vi "From file_test1.vi"() -> (0 "Y subarray":string[](array[string]), 1 "X subarray":string[](array[string]), 2 "Ready?":bool)   [LabVIEW 2021]
uses:
  <vilib>/Utility/file.llb/Read Delimited Spreadsheet (string).vi
panel:
  out "Waveform Graph":dbl[][](graph)
  in  "X data":string(combo)
  out "all rows":string[][](array[string])
  in  "Y data":string(combo)
  in  "Add":bool
  in  "Cancel":bool
  in  "From file (csv)":path caption="file path (dialog if empty)"
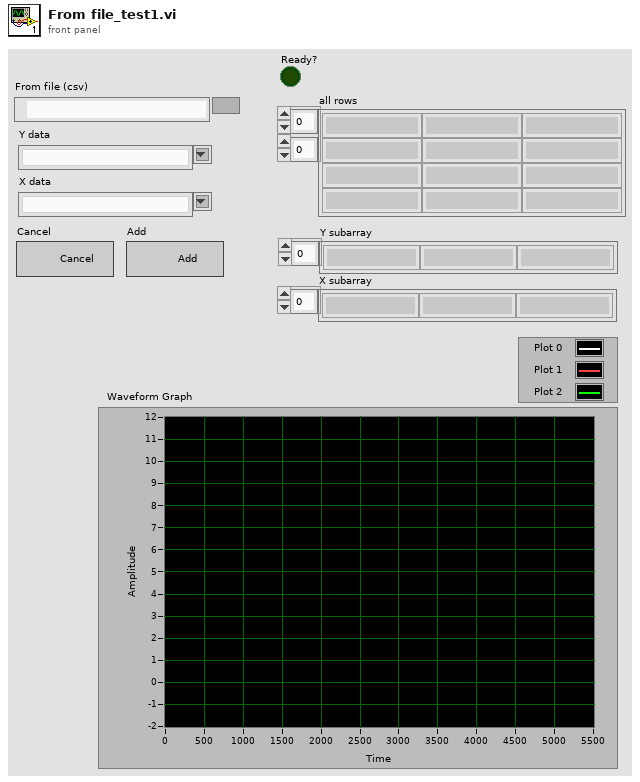
[diagram p1: front panel]
types:
  T1 = enum32{"Invalid", "Standard", "Closed", "Hidden", "Minimized", "Maximized"}
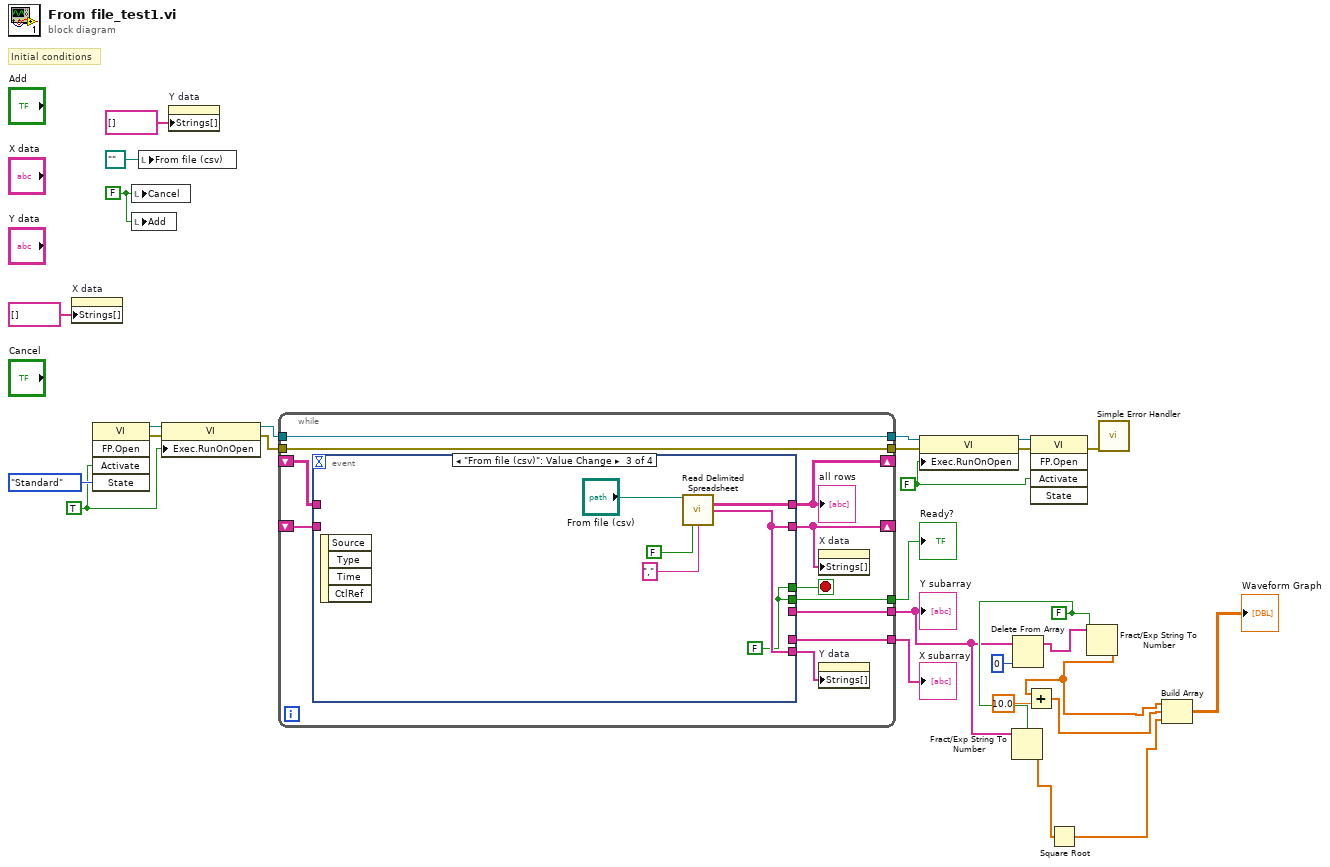
[diagram p0: block diagram]
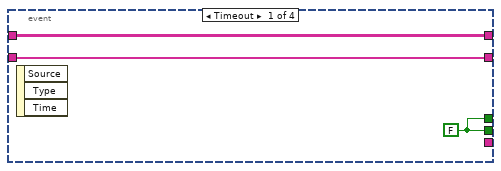
[diagram p2: hidden frame]
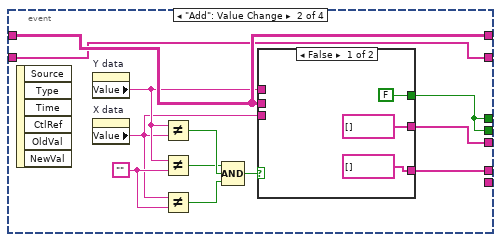
[diagram p3: hidden frame]
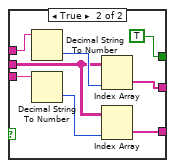
[diagram p4: hidden frame]
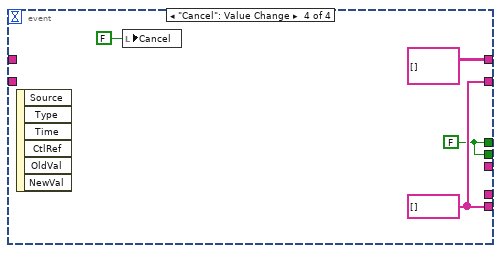
[diagram p5: hidden frame]
diagram:
  w9 = FALSE ("use system decimal point (T)")
  w12 = FALSE ("Activate?")
  w17 = TRUE ("Activate?")
  w27 = FALSE
  # "Initial conditions"
  n1 = property on="X data" class="CmbBox"("Strings[]"=string[] [] ("all rows")) -> ()  [unwired: 2 in, 2 out]
  n2 = invoke class="VI" method="FP.Open"("Activate"=w17, "State"=T1."Standard") -> (reference out=w19:refnum<vi>, error out=w20:errorcluster)  [unwired: 3 in, 3 out]
  n3 = local write "Cancel"(w27) -> ()
  n4 = local write "Add"(w27) -> ()
  n5 = local write "From file (csv)"(path "" ("From file (csv)")) -> ()
  n6 = property class="VI"(reference=w19, error in=w20, "Exec.RunOnOpen"=w17) -> (reference out=w18:refnum<vi>, error out=w21:errorcluster)
  n7 = property on="Y data" class="CmbBox"("Strings[]"=string[] [] ("Strings []")) -> ()  [unwired: 2 in, 2 out]
  n8 = while {
    shift-right: [w36] -> _
    shift-left: _ -> [w38]
    shift-right: [w31] -> _
    shift-left: _ -> [w37]
    tunnel: [w35] -> w1
    tunnel: [w34] -> w5
    tunnel: [w32] -> w26
    tunnel: w21 -> [w29]
    tunnel: w18 -> [w30]
    tunnel: [w30] -> w14
    tunnel: [w29] -> w13
    stop <- w39 stop-if-true
    n9 = event shown="[2] \"From file (csv)\": Value Change" {
      selector: _ -> [_ _ _ _]
      dyn-events: _ -> [_ _ _ _]
      timeout: _ -> [_ _ _ _]
      tunnel: [w42 w49 w68 string[][] [] ("all rows")] -> w36
      tunnel: [w41 w48 w67 w73] -> w31
      tunnel: [w40 w45 w66 w72] -> w39
      tunnel: w38 -> [w42 w49 _ _]
      tunnel: w37 -> [w41 w48 _ _]
      tunnel: [_ w47 _ _] -> w35
      tunnel: [_ w46 _ _] -> w34
      tunnel: [_ _ w67 w73] -> w33
      tunnel: [w40 w45 w66 w72] -> w32
      event Timeout {
        w40 = FALSE
        n10 = event-data() -> ()  [unwired: 1 in, 3 out]
      }
      event "Add": Value Change {
        w51 = ""
        n11 = event-data() -> ()  [unwired: 1 in, 6 out]
        n12 = property on="Y data" class="CmbBox"() -> ("Value"=w44:string)  [unwired: 2 in, 2 out]
        n13 = property on="X data" class="CmbBox"() -> ("Value"=w43:string)  [unwired: 2 in, 2 out]
        n14 = Not Equal?(x=w44, y=w43) -> (x != y?=w53:bool)
        n15 = Not Equal?(x=w44, y=w51) -> (x != y?=w52:bool)
        n16 = Not Equal?(x=w43, y=w51) -> (x != y?=w54:bool)
        n17 = Compound Arithmetic op=AND(w52, w53, w54) -> (w50:bool)
        n18 = case shown="False" w50 {
          tunnel: [FALSE TRUE] -> w45
          tunnel: w49 -> [_ w62]
          tunnel: w44 -> [_ w64]
          tunnel: w43 -> [_ w61]
          tunnel: [string[] [] ("all rows") w59] -> w47
          tunnel: [string[] [] ("all rows") w58] -> w46
          frame False {
          }
          frame True {
            n19 = Decimal String To Number(string=w64) -> (number=w63:i32)  [unwired: 2 in, 1 out]
            n20 = Decimal String To Number(string=w61) -> (number=w60:i32)  [unwired: 2 in, 1 out]
            n21 = Index Array(array=w62, index (col)=w63) -> (element=w59:string[])  [unwired: 1 in]
            n22 = Index Array(array=w62, index (col)=w60) -> (element=w58:string[])  [unwired: 1 in]
          }
        }
      }
      event "From file (csv)": Value Change {
        w66 = FALSE
        n23 = event-data() -> ()  [unwired: 1 in, 4 out]
        n24 = call-poly <vilib>:"Read Delimited Spreadsheet.vi"("file path (dialog if empty)"="From file (csv)", "transpose? (F)"=FALSE, "delimiter (\\t)"="," ("delimiter (\\t)")) -> ("all rows"=w68:string[][], "first row"=w67:string[])  [unwired: 7 in, 4 out]
      }
      event "Cancel": Value Change {
        w72 = FALSE
        w73 = string[] [] ("first row")
        n25 = event-data() -> ()  [unwired: 1 in, 6 out]
        n26 = local write "Cancel"(FALSE) -> ()
      }
    }
    "all rows" <- w36
    n27 = property on="X data" class="CmbBox"("Strings[]"=w31) -> ()  [unwired: 2 in, 2 out]
    n28 = property on="Y data" class="CmbBox"("Strings[]"=w33) -> ()  [unwired: 2 in, 2 out]
  }
  "Y subarray" <- w1
  "X subarray" <- w5
  "Ready?" <- w26
  n29 = property class="VI"(reference=w14, error in=w13, "Exec.RunOnOpen"=w12) -> (reference out=w16:refnum<vi>, error out=w15:errorcluster)
  n30 = Fract/Exp String To Number(use system decimal point (T)=w9, string=w1) -> (number=w7:dbl[])  [unwired: 2 in, 1 out]
  n31 = Delete From Array(array=w1, index=0) -> (array with subset deleted=w10:string[])  [unwired: 1 in, 1 out]
  n32 = invoke class="VI" method="FP.Open"(reference=w16, error in=w15, "Activate"=w12) -> (error out=w22:errorcluster)  [unwired: 2 in, 4 out]
  n33 = Square Root(x=w7) -> (sqrt(x)=w6:dbl[])
  n34 = Fract/Exp String To Number(use system decimal point (T)=w9, string=w10) -> (number=w3:dbl[])  [unwired: 2 in, 1 out]
  n35 = Add(x=w3, y=10.0) -> (x+y=w2:dbl[])
  n36 = call <vilib>:"Simple Error Handler.vi"("error in (no error)"=w22) -> ()  [unwired: 4 in, 5 out]
  n37 = Build Array(w3, w2, w6) -> (→"Waveform Graph":dbl[][])
